vi "FestoCPX.Station.ProdArm.Check.vi"(8 "error in":errorcluster) -> (0 "error out":errorcluster, 1 "NOK":bool, 2 "OK":bool, 3 "Work":bool, 5 "Position":T1)   [LabVIEW 2016]
uses:
  FestoCPX.Station.ProdArmPosition.ctl
  FestoCPX.DI.Signal.ctl
  FestoCPX.DO.Signal.ctl
  FestoCPX.DO.Data.Fglb.vi
  FestoCPX.DI.Data.States.Get.vi
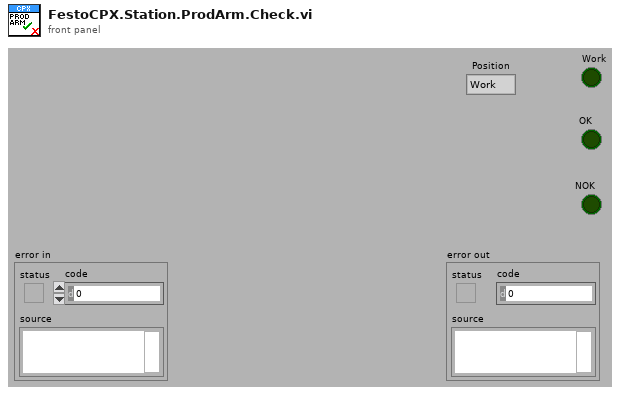
[diagram p1: front panel]
types:
  T1 = typedef "FestoCPX.Station.ProdArmPosition.ctl" = enum16{"Work", "OK", "NOK"}
  T2 = typedef "FestoCPX.DO.Signal.ctl" = enum16{"Safety Reset", "Air Main Valve", "Door Lock", "Button LED Start", "Button LED Stop", "Button LED Control", "Traffic LED Red", "Traffic LED Orange", "Traffic LED Green", "Horn", "Laser Interlock", "Laser Trigger", "Laser Fume Extractor", "Product Suction Gripper Slot 1 A", "Product Suction Gripper Slot 1 B", "Product Suction Gripper Slot 2 A", "Product Suction Gripper Slot 2 B", "Product Suction Gripper Slot 3 A", "Product Suction Gripper Slot 3 B", "Product Suction Gripper Slot 4 A", "Product Suction Gripper Slot 4 B", "Product Suction Gripper Final A", "Product Suction Gripper Final B", "Lamp", "Q1 Product Move Work", "Q1 Product Move Home", "Q2 Table Turn Work", "Q2 Table Turn Home", "Q3 Product Lift A", "Q3 Product Lift B", "Q4 Product Arm OK", "Q4 Product Arm NOK", "Q5 Product Arm Work", "Q6 Product BlowOut A", "Q6 Product BlowOut B"}
  T3 = typedef "FestoCPX.DI.Signal.ctl" = enum16{"S.C. Emergency Stop", "S.C. Side Door Close", "S.C. Front Door Close", "S.C. Front Door Secured", "Button Start", "Button Stop", "Button Control", "Product Move Home", "Product Move Work", "Table Position", "Table Lock", "Product Lift A Home", "Product Lift B Home", "Product Arm OK", "Product Arm NOK", "Product Arm Work", "Revolver ID 1", "Revolver ID 2", "Revolver ID 3", "Revolver ID 4", "Revolver ID 5", "Air Pressure Inside", "Air Pressure Inlet", "Product Slot 1 A Present", "Product Slot 1 B Present", "Product Slot 2 A Present", "Product Slot 2 B Present", "Product Slot 3 A Present", "Product Slot 3 B Present", "Product Slot 4 A Present", "Product Slot 4 B Present", "Product Final A Present", "Product Final B Present", "Product Output A Present", "Product Output B Present", "Product Container OK Present", "Product Container NOK Present", "Fork ID 1", "Fork ID 2"}
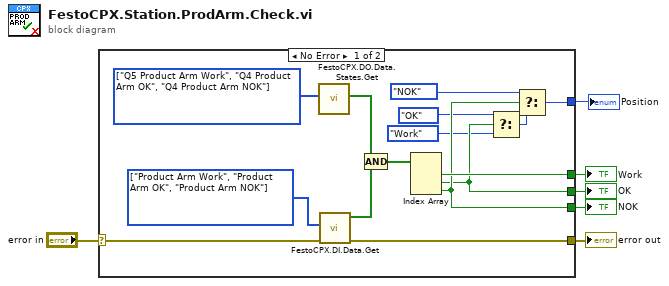
[diagram p0: block diagram]
diagram:
  n1 = case shown="No Error" "error in" {
    selector: "error in" -> [w18 w22]
    tunnel: [w17 w22] -> w6
    tunnel: [w13 _] -> w4
    tunnel: [w15 _] -> w3
    tunnel: [w16 _] -> w2
    tunnel: [w9 _] -> w1
    frame No Error {
      w20 = T2[] [enum."Q5 Product Arm Work", enum."Q4 Product Arm OK", enum."Q4 Product Arm NOK"] items=["Safety Reset", "Air Main Valve", "Door Lock", "Button LED Start", "Button LED Stop", "Button LED Control", "Traffic LED Red", "Traffic LED Orange", "Traffic LED Green", "Horn", "Laser Interlock", "Laser Trigger", "Laser Fume Extractor", "Product Suction Gripper Slot 1 A", "Product Suction Gripper Slot 1 B", "Product Suction Gripper Slot 2 A", "Product Suction Gripper Slot 2 B", "Product Suction Gripper Slot 3 A", "Product Suction Gripper Slot 3 B", "Product Suction Gripper Slot 4 A", "Product Suction Gripper Slot 4 B", "Product Suction Gripper Final A", "Product Suction Gripper Final B", "Lamp", "Q1 Product Move Work", "Q1 Product Move Home", "Q2 Table Turn Work", "Q2 Table Turn Home", "Q3 Product Lift A", "Q3 Product Lift B", "Q4 Product Arm OK", "Q4 Product Arm NOK", "Q5 Product Arm Work", "Q6 Product BlowOut A", "Q6 Product BlowOut B"] ("CPX.DO")
      w21 = T3[] [enum."Product Arm Work", enum."Product Arm OK", enum."Product Arm NOK"] items=["S.C. Emergency Stop", "S.C. Side Door Close", "S.C. Front Door Close", "S.C. Front Door Secured", "Button Start", "Button Stop", "Button Control", "Product Move Home", "Product Move Work", "Table Position", "Table Lock", "Product Lift A Home", "Product Lift B Home", "Product Arm OK", "Product Arm NOK", "Product Arm Work", "Revolver ID 1", "Revolver ID 2", "Revolver ID 3", "Revolver ID 4", "Revolver ID 5", "Air Pressure Inside", "Air Pressure Inlet", "Product Slot 1 A Present", "Product Slot 1 B Present", "Product Slot 2 A Present", "Product Slot 2 B Present", "Product Slot 3 A Present", "Product Slot 3 B Present", "Product Slot 4 A Present", "Product Slot 4 B Present", "Product Final A Present", "Product Final B Present", "Product Output A Present", "Product Output B Present", "Product Container OK Present", "Product Container NOK Present", "Fork ID 1", "Fork ID 2"]
      n2 = call "FestoCPX.DO.Data.States.Get.vi"("CPX.DO"=w20) -> ("State"=w8:bool[])  [unwired: 9 in, 1 out]
      n3 = call-poly "FestoCPX.DI.Data.Get.vi"("error in (no error)"=w18, "CPX.DI"=w21) -> ("error out"=w17:errorcluster, "State"=w7:bool[])  [unwired: 5 in, 3 out]
      n4 = Compound Arithmetic op=AND(w8, w7) -> (w19:bool[])
      n5 = Index Array(array=w19) -> (element #1=w16:bool, element #2=w13:bool, element #3=w15:bool)  [unwired: 3 in]
      n6 = Select(t=FestoCPX.Station.ProdArmPosition."OK" ("Product Arm Position"), s=w13, f=FestoCPX.Station.ProdArmPosition."Work" ("Product Arm Position")) -> (s? t:f=w10:T1)
      n7 = Select(t=FestoCPX.Station.ProdArmPosition."NOK" ("Product Arm Position"), s=w15, f=w10) -> (s? t:f=w9:T1)
    }
    frame Error {
    }
  }
  "error out" <- w6
  "OK" <- w4
  "NOK" <- w3
  "Work" <- w2
  "Position" <- w1
